vi "Init Actor.vi"() -> (2 "Actor":refnum<class "Actor.lvclass">)   [LabVIEW 2020, in "jettl.lvlib" / "Base jettl Actor.lvlib"]
uses:
  Base jettl Actor.lvlib
  Base Actor/Base Actor.lvlib
  Actor/Actor.lvclass
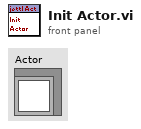
[diagram p1: front panel]
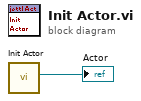
[diagram p0: block diagram]
diagram:
  n1 = call "Init Actor.vi"() -> ("Actor"=→"Actor":refnum<class "Actor.lvclass">)  [unwired: 11 in]
